vi "Configure Marker Search.vi"(7 "Marker Search (Max Peak)":T1, 8 "error in (no error)":errorcluster, 10 "Marker Number (1)":u32=1 min=1, 11 "SA-ESA in":refnum<class "SA-ESA.lvclass">) -> (0 "error out":errorcluster, 3 "SA-ESA out":refnum<class "SA-ESA.lvclass">)   [LabVIEW 2020, in "SA-ESA.lvclass"]
uses:
  SA-ESA.lvclass
  C:/Sandbox/RF Bench/Source Code/WiSpry Test Framework/Instruments/Instrument.lvclass
  Controls/Marker Search.ctl
  Instrument.lvclass/Instrument.ctl
  Spectrum Analyzer.lvclass
  Instrument.lvclass
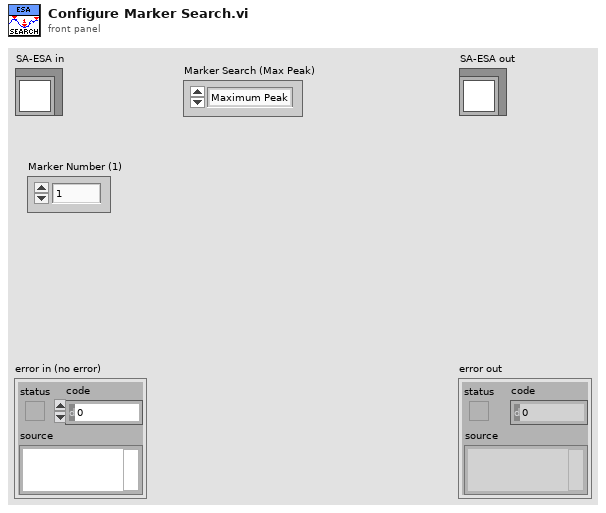
[diagram p1: front panel]
types:
  T1 = typedef "Spectrum Analyzer.lvclass/Marker Search.ctl" = enum16{"Maximum Peak", "Maximum Next", "Maximum Right", "Maximum Left", "Minimum Peak", "Minimum Next", "Minimum Right", "Minimum Left"}
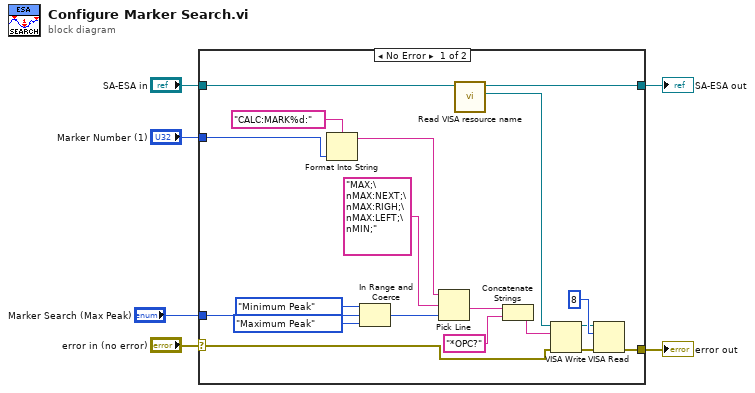
[diagram p0: block diagram]
diagram:
  n1 = case shown="No Error" "error in (no error)" {
    selector: "error in (no error)" -> [w13 w26]
    tunnel: "SA-ESA in" -> [w17 w27]
    tunnel: "Marker Number (1)" -> [w24 _]
    tunnel: "Marker Search (Max Peak)" -> [w21 _]
    tunnel: [w8 w26] -> w1
    tunnel: [w7 w27] -> w2
    frame No Error {
      n2 = Format Into String(format string="CALC:MARK%d:", w24) -> (resulting string=w23:string)  [unwired: 2 in, 1 out]
      n3 = In Range and Coerce(upper limit=Marker_Search."Minimum Peak", x=w21, lower limit=Marker_Search."Maximum Peak") -> (coerced(x)=w20:T1)  [unwired: 1 out]
      n4 = Pick Line(string ("")=w23, multi-line string="MAX;\nMAX:NEXT;\nMAX:RIGH;\nMAX:LEFT;\nMIN;", line index=w20) -> (output string=w16:string)
      n5 = call "Read VISA resource name.vi"("Instrument in"=w17) -> ("VISA resource name"=w12:refnum<visa-resource-name>, "Instrument out"=w7:refnum<class "SA-ESA.lvclass">)  [unwired: 9 in]
      n6 = Concatenate Strings(w16, "*OPC?" ("string")) -> (w11:string)
      n7 = VISA Write(VISA resource name=w12, write buffer=w11, error in (no error)=w13) -> (VISA resource name out=w10:refnum<visa-resource-name>, error out=w9:errorcluster)  [unwired: 1 out]
      n8 = VISA Read(VISA resource name=w10, byte count=u32 8, error in (no error)=w9) -> (error out=w8:errorcluster)  [unwired: 3 out]
    }
    frame Error {
    }
  }
  "error out" <- w1
  "SA-ESA out" <- w2
